vi "Send Configure Sparse Marker [SM].vi"(4 "Indexes Array":i64[](array[numeric]) caption="indexes array", 5 "Waveform Handle":i32 caption="waveform handle" format="%.0g", 6 "Number Indexes":i64 caption="number indexes" format="%.0g", 7 "Message Priority (Normal)":T1=enum."Normal", 8 "error in (no error)":errorcluster, 9 "Destination Terminal (None)":string(combo) caption="destination terminal (None)", 10 "Marker Name (\"\")":string caption="marker name (\"\")", 11 "Message Enqueuer":refnum<class "Message Enqueuer.lvclass">) -> (0 "error out":errorcluster, 3 "Message Enqueuer out":refnum<class "Message Enqueuer.lvclass">)   [LabVIEW 2013, in "CS++Fgen.lvlib" / "Configure Sparse Marker [SM] Msg.lvclass"]
doc: "This VI sends the message to an actor."
uses:
  Configure Sparse Marker [SM] Msg.lvclass
  <vilib>/ActorFramework/Message Enqueuer/Message Enqueuer.lvclass
  <vilib>/ActorFramework/Message Enqueuer/Message Priority.ctl
  Configure Sparse Marker [SM] Msg.lvclass/Configure Sparse Marker [SM] Msg.ctl
  <vilib>/ActorFramework/Message Enqueuer/Message Enqueuer.lvclass/Message Enqueuer.ctl
  <vilib>/ActorFramework/Message Priority Queue/Priority Enqueue.vi
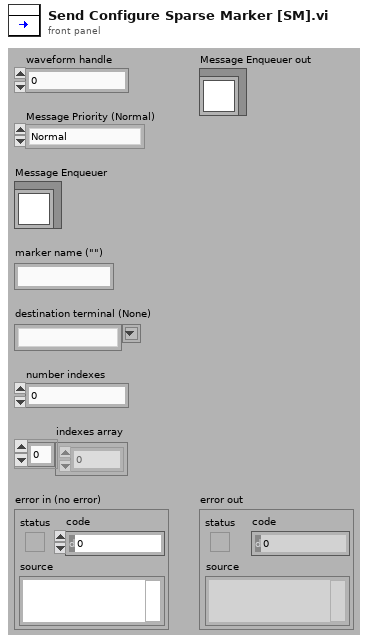
[diagram p1: front panel]
types:
  T1 = typedef "Actor Framework.lvlib/Message Enqueuer.lvclass/Message Priority.ctl" = enum16{"Low", "Normal", "High"}
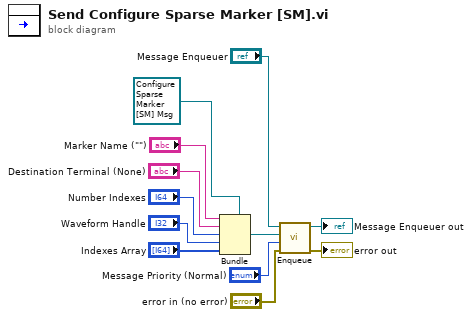
[diagram p0: block diagram]
diagram:
  n1 = Bundle(cluster=refnum<class "Configure Sparse Marker [SM] Msg.lvclass"> refnum ("Object"), "Marker Name (\"\")", "Destination Terminal (None)", "Number Indexes", "Waveform Handle", "Indexes Array") -> (w8:refnum<class "Configure Sparse Marker [SM] Msg.lvclass">)
  n2 = call <vilib>:"Enqueue.vi"("error in (no error)"="error in (no error)", "Message Priority (Normal)"="Message Priority (Normal)", "Message"=w8, "Message Enqueuer in"="Message Enqueuer") -> ("error out"=→"error out":errorcluster, "Message Enqueuer out"=→"Message Enqueuer out":refnum<class "Message Enqueuer.lvclass">)  [unwired: 6 in]
